vi "Set Mobile Platform.vi"(8 "error in (no error)":errorcluster, 10 "KUKA youBot platform in":refnum<class "NI_Robotics_KUKA youBot Platform.lvclass">, 11 "KUKA youBot host in":refnum<class "NI_Robotics_KUKA youBot Host Interface.lvclass">) -> (0 "error out":errorcluster, 3 "KUKA youBot host out":refnum<class "NI_Robotics_KUKA youBot Host Interface.lvclass">)   [LabVIEW 2017, in "NI_Robotics_KUKA youBot Host.lvlib" / "NI_Robotics_KUKA youBot Host Interface.lvclass"]
uses:
  <vilib>/robotics/KUKA youBot/Host Interface/NI_Robotics_KUKA youBot Host Interface.lvclass
  <vilib>/robotics/KUKA youBot/Basic Device/Mobile Platform/NI_Robotics_KUKA youBot Platform.lvclass
  <vilib>/robotics/KUKA youBot/Host Interface/NI_Robotics_KUKA youBot Host Interface.lvclass/NI_Robotics_KUKA youBot Host Interface.ctl
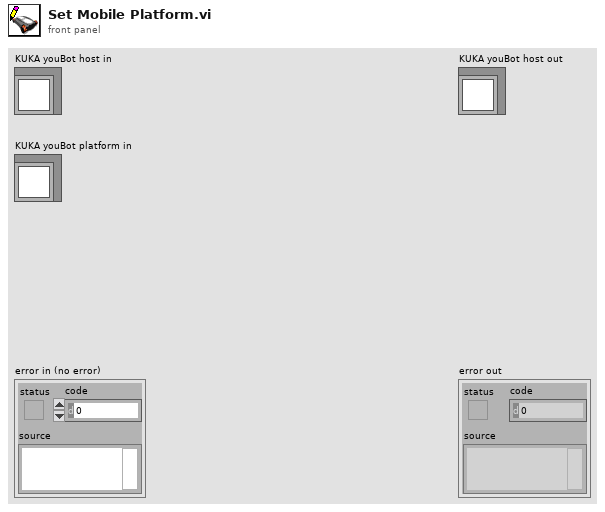
[diagram p1: front panel]
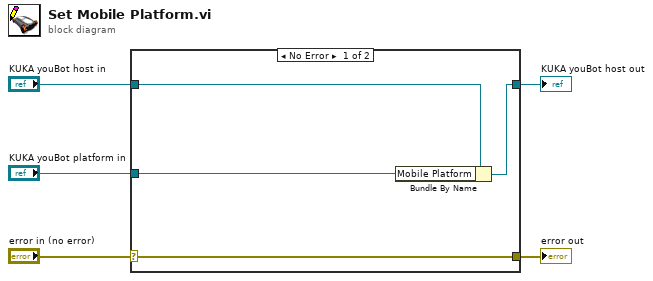
[diagram p0: block diagram]
diagram:
  n1 = case shown="No Error" "error in (no error)" {
    selector: "error in (no error)" -> [w9 w10]
    tunnel: [w9 w10] -> w4
    tunnel: [w7 w11] -> w2
    tunnel: "KUKA youBot host in" -> [w8 w11]
    tunnel: "KUKA youBot platform in" -> [w6 _]
    frame No Error {
      n2 = Bundle By Name(cluster=w8, "Mobile Platform"=w6) -> (w7:refnum<class "NI_Robotics_KUKA youBot Host Interface.lvclass">)
    }
    frame Error {
    }
  }
  "error out" <- w4
  "KUKA youBot host out" <- w2
